vi "refgen_inner.vi"(8 "queue in":refnum<queue>, 11 "Qube":refnum<class "System.lvclass">) -> (3 "Qube":refnum<class "System.lvclass">)   [LabVIEW 2021, in "System.lvclass"]
uses:
  System.lvclass
  System.lvclass/System.ctl
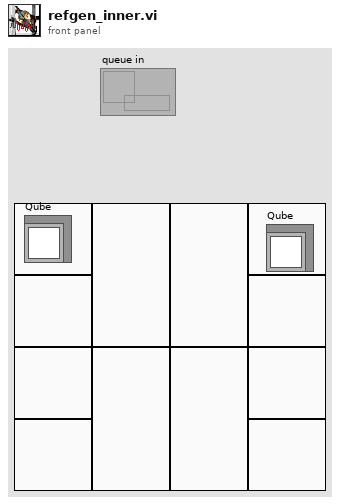
[diagram p1: front panel]
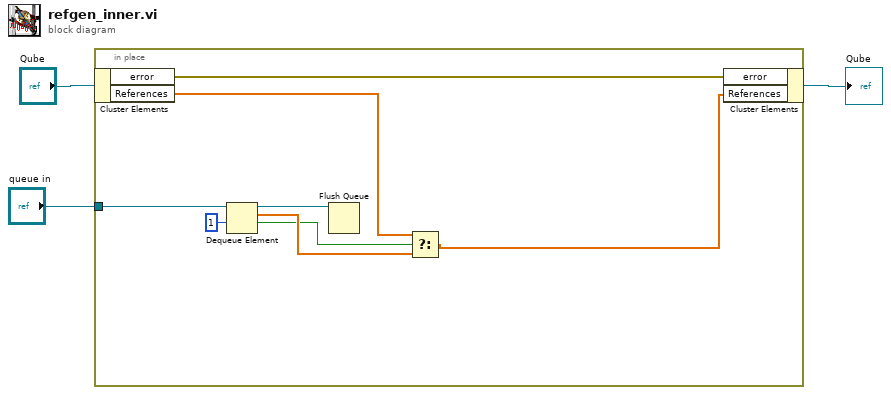
[diagram p0: block diagram]
diagram:
  n1 = in-place {
    in-place-border: "queue in" -> [w9]
    n2 = in-place-cluster #1("Qube") -> ("error"=w11:errorcluster, "References"=w10:dbl[])
    n3 = Dequeue Element(queue=w9, timeout in ms (-1)=1) -> (queue out=w7:refnum<queue>, element=w8:dbl[], timed out?=w5:bool)  [unwired: 1 in, 1 out]
    n4 = Flush Queue(queue=w7) -> ()  [unwired: 1 in, 3 out]
    n5 = Select(t=w10, s=w5, f=w8) -> (s? t:f=w4:dbl[])
    n6 = in-place-cluster #1("error"=w11, "References"=w4) -> (→"Qube":refnum<class "System.lvclass">)
  }
